vi "close file and backup.vi"(8 "error in":errorcluster, 10 "backup directory":path, 11 "tdms file in":refnum<k34>) -> (0 "error out":errorcluster)   [LabVIEW 2013, in "TDMS datalogger runtime.lvclass"]
uses:
  TDMS datalogger runtime.lvclass
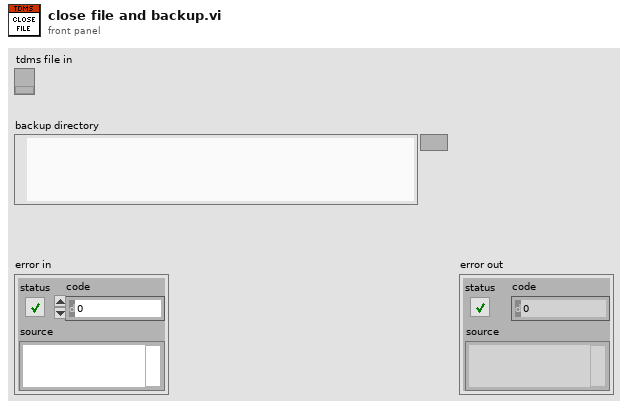
[diagram p1: front panel]
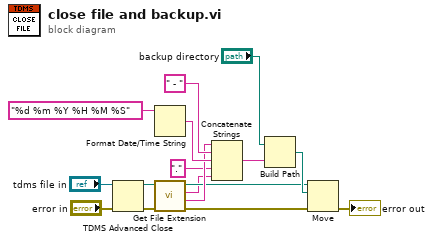
[diagram p0: block diagram]
diagram:
  n1 = TDMS Advanced Close(8:"error in", 11:"tdms file in") -> (0:w11:errorcluster, 3:w12:path)  [unwired: 2 in]
  n2 = Format Date/Time String(time format string (%c)="%d %m %Y %H %M %S") -> (date/time string=w13:string)  [unwired: 2 out]
  n3 = call <vilib>:"Get File Extension.vi"("error in (no error)"=w11, "file"=w12) -> ("error out"=w4:errorcluster, "filename without extension"=w10:string, "lowercase file extension"=w3:string, "dup file"=w5:path)  [unwired: 6 in]
  n4 = Concatenate Strings(w10, " - " ("string"), w13, "." ("string"), w3) -> (w1:string)
  n5 = Build Path(base path="backup directory", name or relative path=w1) -> (appended path=w6:path)
  n6 = Move(source path=w5, error in=w4, 10:w6) -> (error out=→"error out":errorcluster)  [unwired: 2 in, 2 out]
